vi "TDT Ramp Test.vi"() -> ()   [LabVIEW 2015]
uses:
  TDT VIs/TDT-Signal Bank Action.ctl
  <vilib>/Analysis/NI_AALBase.lvlib
panel:
  in  "stop":bool
  in  "Ramp (ms)":dbl=10.0
  in  "Freq (Hz)":dbl=500.0
  in  "Frame size (s)":dbl=0.05
  in  "Fs (Hz)":dbl=100000.0
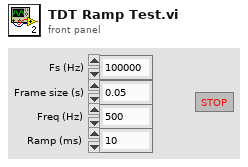
[diagram p1: front panel]
types:
  T1 = typedef "TDT-Signal Bank Action.ctl" = enum16{"Init", "Write", "Read", "Rewrite", "Reset", "Recycle", "Ramp up", "Ramp down", "Zero"}
  T2 = typedef "TDT-Device Config.ctl" = cluster{"Output":T3, "Input":T5}
  T3 = typedef "TDT-Output source.ctl" = cluster{"Device":T4, "Num":i32}
  T4 = typedef "TDT-Device ID.ctl" = enum16{"None", "PA5", "RP2", "RL2", "RA16", "RV8", "RX5", "RX6", "RX7", "RX8", "RZ2", "RZ5", "RZ6"}
  T5 = typedef "TDT-Input source.ctl" = enum16{"Front Panel", "RA4LI", "RA16LI"}
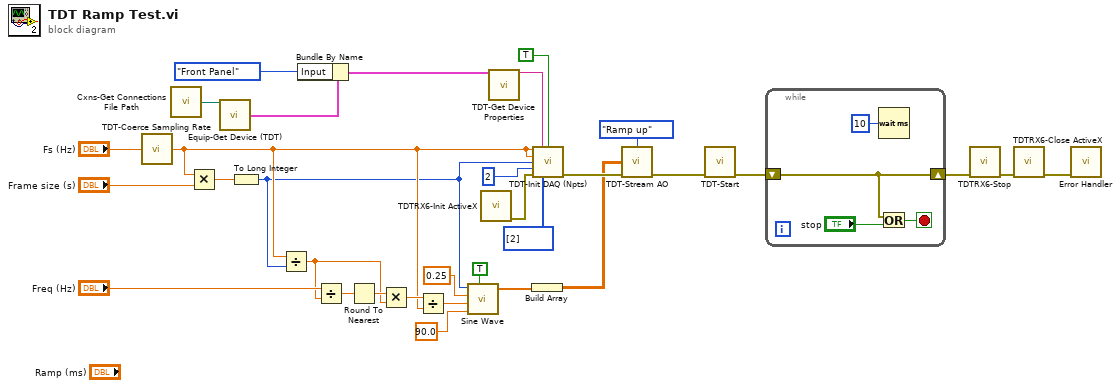
[diagram p0: block diagram]
diagram:
  n1 = call "TDT-Coerce Sampling Rate.vi"("Fs (Hz)"="Fs (Hz)") -> ("Coerced"=w7:dbl)
  n2 = call "Cxns-Get Connections File Path.vi"() -> ("Path Out"=w29:path)  [unwired: 1 in]
  n3 = Multiply(x=w7, y="Frame size (s)") -> (x*y=w31:dbl)
  n4 = call "Equip-Get Device (TDT).vi"("Path In"=w29) -> ("TDT-Device Config"=w30:T2)  [unwired: 12 in, 2 out]
  n5 = To Long Integer(number=w31) -> (32bit integer=w6:i32)
  n6 = Divide(x=w7, y=w6) -> (x/y=w9:dbl)
  n7 = Bundle By Name(cluster=w30, "Input"=enum16{"Front Panel", "RA4LI", "RA16LI"}."Front Panel") -> (w27:T2)
  n8 = Divide(x="Freq (Hz)", y=w9) -> (x/y=w11:dbl)
  n9 = Round To Nearest(number=w11) -> (nearest integer value=w12:dbl)
  n10 = Multiply(x=w12, y=w9) -> (x*y=w8:dbl)
  n11 = Divide(x=w8, y=w7) -> (x/y=w4:dbl)
  n12 = call <vilib>:"Sine Wave.vi"("samples"=w6, "amplitude"=0.25, "frequency"=w4, "phase in"=90.0, "reset phase"=TRUE) -> ("sine wave"=w2:dbl[])  [unwired: 2 out]
  n13 = call "TDTRX6-Init ActiveX.vi"() -> ("error out"=w16:errorcluster)  [unwired: 14 in, 1 out]
  n14 = call "TDT-Get Device Properties.vi"("TDT-Device Config"=w27) -> ("Circuit File"=w26:string)  [unwired: 9 in, 5 out]
  n15 = Build Array(w2) -> (w18:dbl[][])
  n16 = call "TDT-Init DAQ (Npts).vi"("AO Fs (Hz)"=w7, "Circuit"=w26, "AI only"=TRUE, "AI Fs (Hz)"=w7, "Num AO Pts"=w6, "Num AO Buffers"=2, "error in (no error)"=w16, "AO Channels"=i32[] [2]) -> ("error out"=w21:errorcluster)  [unwired: 3 in, 4 out]
  n17 = call "TDT-Stream AO.vi"("Action"=TDT-Signal_Bank_Action."Ramp up", "Output array"=w18, "error in (no error)"=w21) -> ("error out"=w14:errorcluster)  [unwired: 12 in]
  n18 = call "TDT-Start.vi"("error in (no error)"=w14) -> ("error out"=w13:errorcluster)  [unwired: 6 in]
  n19 = while {
    shift-right: [w33] -> w20
    shift-left: w13 -> [w33]
    stop <- w34 stop-if-true
    n20 = Wait (ms)(milliseconds to wait=u32 10) -> ()  [unwired: 1 out]
    n21 = Or(x=w33, y="stop") -> (x .or. y?=w34:bool)
  }
  n22 = call "TDTRX6-Stop.vi"("error in (no error)"=w20) -> ("error out"=w19:errorcluster)  [unwired: 14 in]
  n23 = call "TDTRX6-Close ActiveX.vi"("error in (no error)"=w19) -> ("error out"=w15:errorcluster)  [unwired: 14 in]
  n24 = call "Error Handler.vi"("error in (no error)"=w15) -> ()  [unwired: 13 in, 2 out]
